vi "saveEvent.vi"(8 "error in (no error)":errorcluster, 11 "PixelflySettings in":refnum<class "PixelflySettings.lvclass">) -> (0 "error out":errorcluster, 3 "PixelflySettings out":refnum<class "PixelflySettings.lvclass">)   [LabVIEW 2009, in "Tools.lvlib" / "Settings.lvlib" / "PixelflySettings.lvclass"]
uses:
  PixelflySettings.lvclass
  PixelflySettings.lvclass/PixelflySettings.ctl
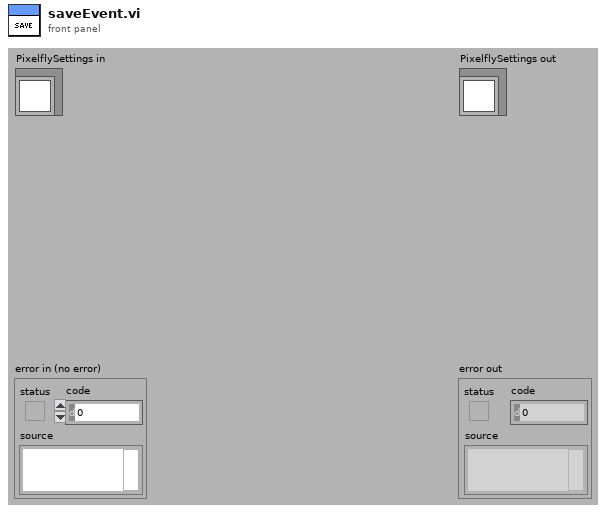
[diagram p1: front panel]
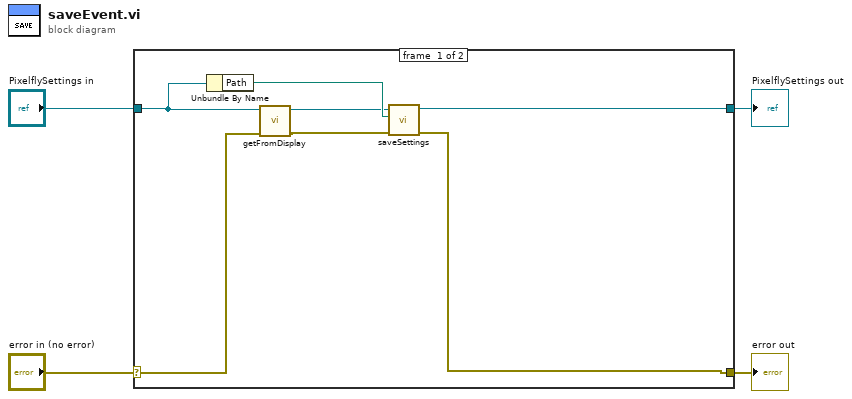
[diagram p0: block diagram]
diagram:
  n1 = case shown="No Error" "error in (no error)" {
    selector: "error in (no error)" -> [w5 w13]
    tunnel: [w9 w13] -> w3
    tunnel: [w10 w12] -> w1
    tunnel: "PixelflySettings in" -> [w8 w12]
    frame #0 {
      n2 = Unbundle By Name(w8) -> ("Path"=w11:path)
      n3 = call "getFromDisplay.vi"("error in (no error)"=w5, "PixelflySettings in"=w8) -> ("error out"=w6:errorcluster, "PixelflySettings out"=w7:refnum<class "PixelflySettings.lvclass">)  [unwired: 8 in]
      n4 = call-dynamic "saveSettings.vi"("error in (no error)"=w6, "Path"=w11, "PixelflySettings in"=w7) -> ("error out"=w9:errorcluster, "PixelflySettings out"=w10:refnum<class "PixelflySettings.lvclass">)  [unwired: 7 in]
    }
    frame #1 {
    }
  }
  "error out" <- w3
  "PixelflySettings out" <- w1
